vi "ziExample-ReadSingleValue.vi"(0 "Address":string="DEV", 1 "oscs/*/freq":dbl=12345.0 caption="Frequency (Hz)" format="%#_6p", 2 "demods/0/timeconstant":dbl=0.001 caption="TC (s)" format="%#_6p", 3 "phaseshift":dbl=12.0 caption="Phase (deg)" format="%#_6p", 4 "demods/0/harmonic":dbl caption="Harmonic", 5 "settingspath":string caption="Settings Path", 7 "Load":bool, 8 "Save":bool) -> (20 "Time since last boot (s)":dbl, 21 "R (Vrms)":dbl format="%#_4g", 22 "Theta (rad)":dbl, 24 "Selected Device":string)   [LabVIEW 2009]
doc: "Control a Zurich instrument device via the LabOne Labview API. \nRequirements: Zurich Instruments MFLI, HF2 or UHFLI \nExample from the Getting Started guide: A single demodulator value is read and unbundled read timestamp, X and Y.\n\n© Zurich Instruments AG, www.zhinst.com"
uses:
  <instrlib>/Zurich Instruments LabOne/Public/Data/ziTypeDemodSampleSingle.ctl
  <instrlib>/Zurich Instruments LabOne/Public/Configure/ziSetValueDoubleArray.vi
  <instrlib>/Zurich Instruments LabOne/Public/Configure/ziGetValueDouble.vi
  <instrlib>/Zurich Instruments LabOne/Public/Utility/ziTicksToS_single.vi
  <instrlib>/Zurich Instruments LabOne/Public/Configure/ziGetValueDemodSampleEx.vi
  <instrlib>/Zurich Instruments LabOne/Zurich Instruments LabOne.lvlib
panel:
  in  "stop":bool
  out "Demod Sample Out":T1={"Timestamps (ticks)"=0, "X (Vrms)"=nan, "Y (Vrms)"=nan, "Osc Phase (deg)"=nan, "Freq (Hz)"=nan, "DIO"=0, "AuxIn0 (V)"=nan, "AuxIn1 (V)"=nan, "Trigger"=0}
  out "Error Out":errorcluster
  # "This example describes how ziGetValueDemodSample.vi can be used"
  # "ziExample-ReadSingleValue.vi\nRequirements: HF2, UHFLI or MFLI\nsee block diagram for VI description"
  # "Settings"
  # "Unbundled output"
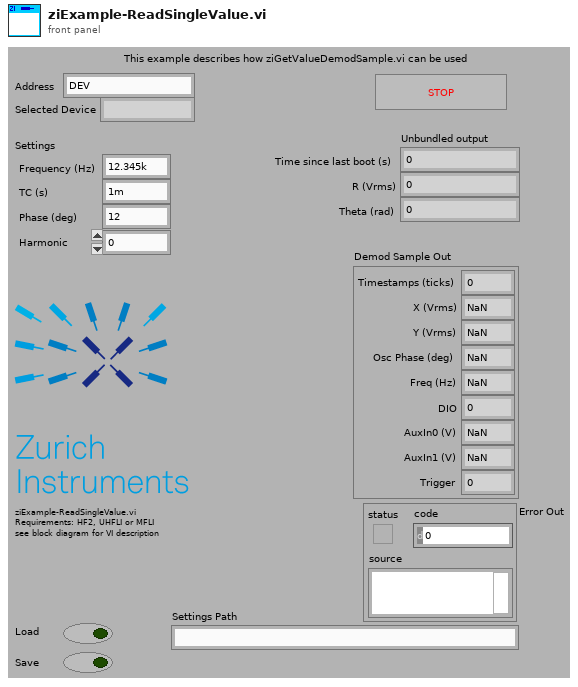
[diagram p1: front panel]
types:
  T1 = typedef "Zurich Instruments LabOne.lvlib/ziTypeDemodSampleSingle.ctl" = cluster{"Timestamps (ticks)":u64, "X (Vrms)":dbl, "Y (Vrms)":dbl, "Osc Phase (deg)":dbl, "Freq (Hz)":dbl, "DIO":u32, "AuxIn0 (V)":dbl, "AuxIn1 (V)":dbl, "Trigger":u32}
  T2 = typedef "Zurich Instruments LabOne.lvlib/ziTypeHandle.ctl" = cluster{"handleValid":bool, "Conn":u64, "Path Prefix":string, "Handle":u64, "Connected":bool, "Clockbase(s)":dbl}
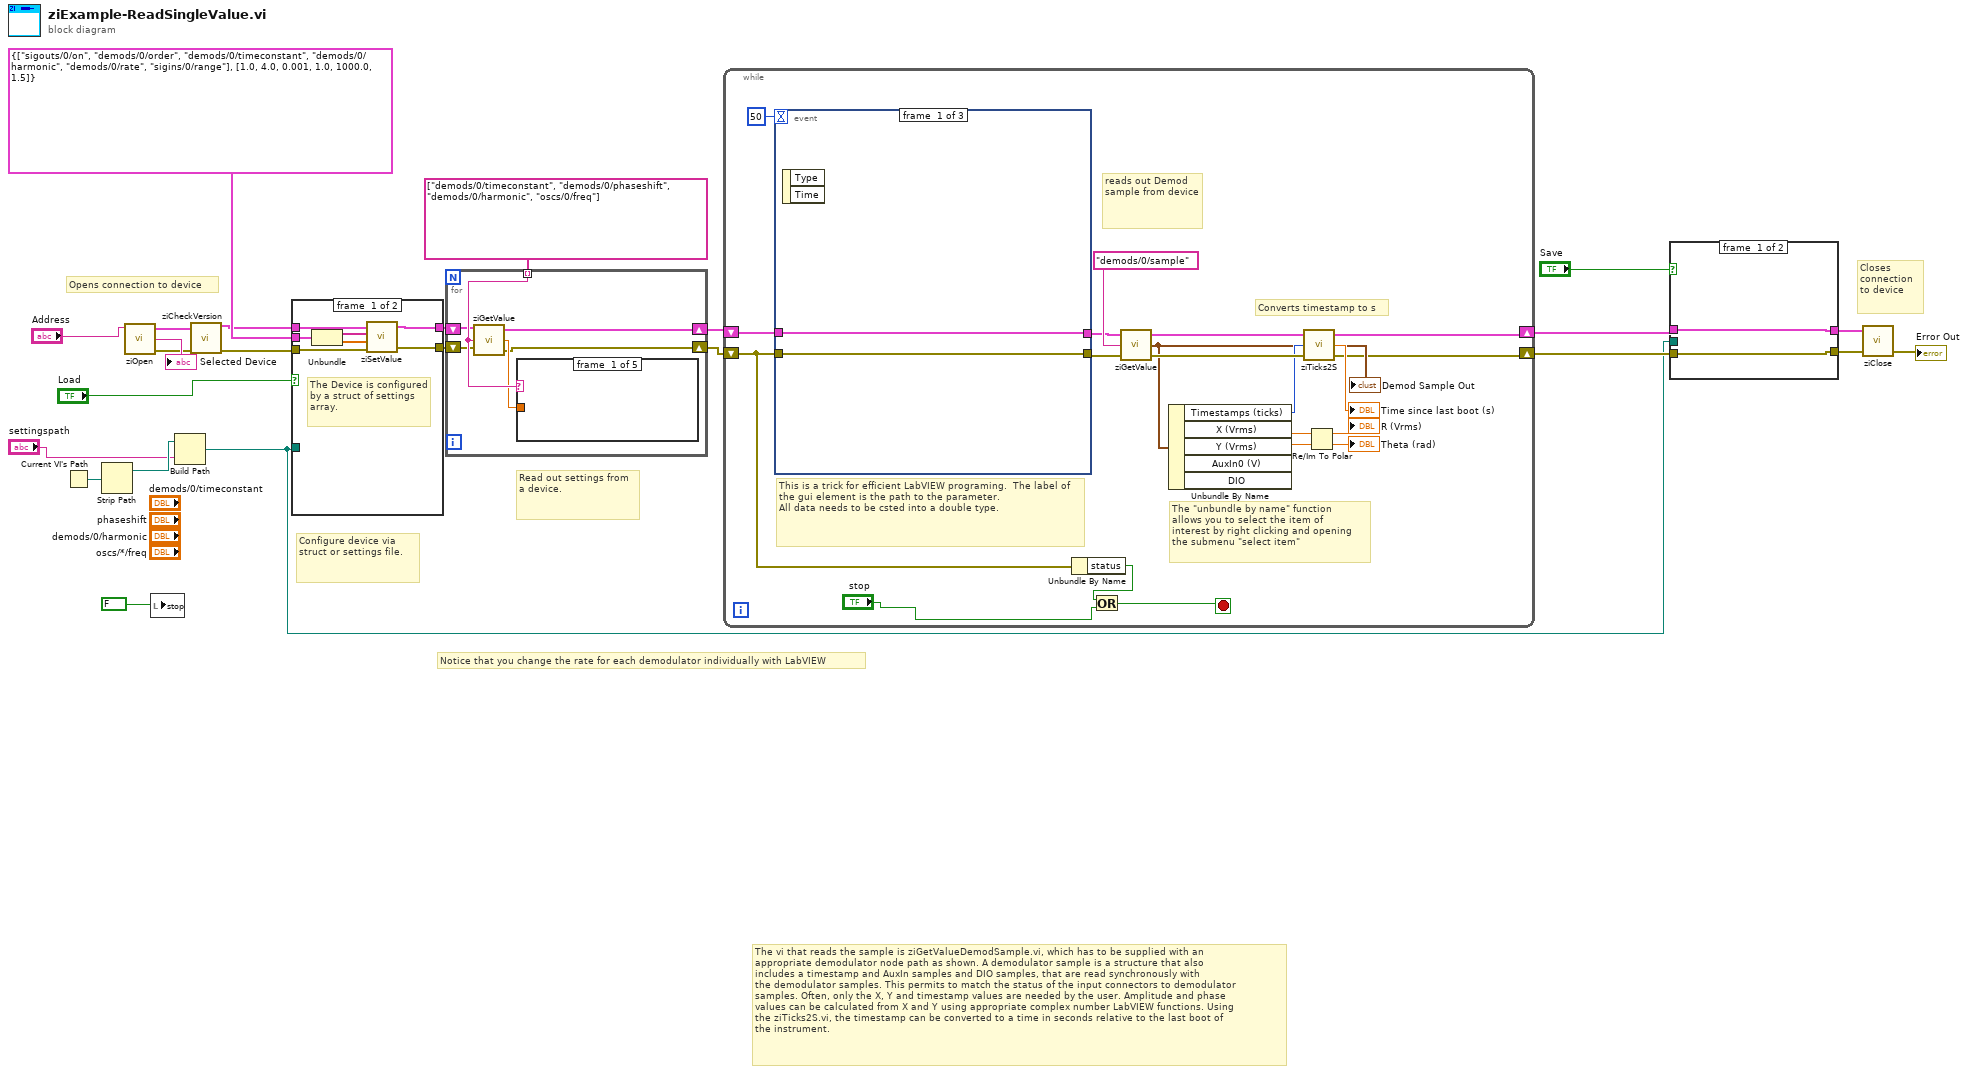
[diagram p0: block diagram]
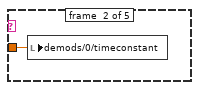
[diagram p2: hidden frame]
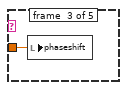
[diagram p3: hidden frame]
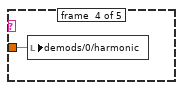
[diagram p4: hidden frame]
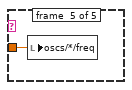
[diagram p5: hidden frame]
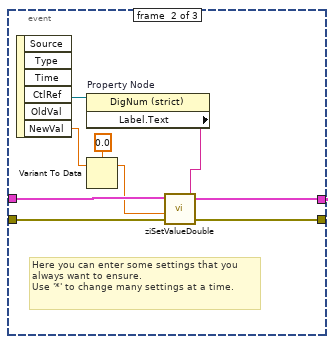
[diagram p6: hidden frame]
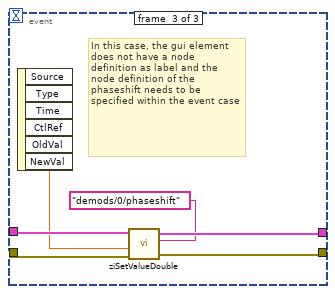
[diagram p7: hidden frame]
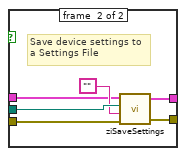
[diagram p8: hidden frame]
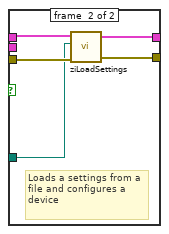
[diagram p9: hidden frame]
diagram:
  # "Closes connection to device"
  # "Opens connection to device"
  # "Read out settings from a device."
  # "Configure device via struct or settings file."
  # "Notice that you change the rate for each demodulator individually with LabVIEW"
  # "The vi that reads the sample is ziGetValueDemodSample.vi, which has to be supplied with an \nappropriate demodulator node path as shown. A demodulator sample is a structure that also \nincludes a timestamp and AuxIn samples and DIO samples, that are read synchronously with \nthe demodulator samples. This permits to match the status of the input connectors to demodulator \nsamples. Often, only the X, Y and timestamp values are needed by the user. Amplitude and phase\nvalues can be calculated from X and Y using appropriate complex number LabVIEW functions. Using \nthe ziTicks2S.vi, the timestamp can be converted to a time in seconds relative to the last boot of \nthe instrument."
  n1 = Current VI's Path() -> (path=w9:path)
  n2 = Strip Path(path=w9) -> (stripped path=w8:path)  [unwired: 1 out]
  n3 = call <instrlib>:"ziOpen.vi"("Address"="Address") -> ("Error Out"=w4:errorcluster, "Selected Device"=→"Selected Device":string, "HandleOut"=w5:T2)  [unwired: 3 in]
  n4 = local write "stop"(FALSE) -> ()
  n5 = Build Path(base path=w8, name or relative path="settingspath") -> (appended path=w6:path)
  n6 = call <instrlib>:"ziCheckVersion.vi"("Handle In"=w5, "Error In"=w4) -> ("Handle Out"=w2:T2, "Error Out"=w3:errorcluster)  [unwired: 11 in, 1 out]
  n7 = case shown="True" "Load" {
    tunnel: w3 -> [w31 w36]
    tunnel: w2 -> [w30 w33]
    tunnel: [w29 w34] -> w14
    tunnel: [w28 w35] -> w13
    tunnel: cluster{string[], dbl[]} {["sigouts/0/on", "demods/0/order", "demods/0/timeconstant", "demods/0/harmonic", "demods/0/rate", "sigins/0/range"], [1.0, 4.0, 0.001, 1.0, 1000.0, 1.5]} -> [w27 _]
    tunnel: w6 -> [_ w32]
    frame #0 {
      # "The Device is configured by a struct of settings array."
      n8 = Unbundle(w27) -> (w26:string[], w25:dbl[])
      n9 = call-poly <instrlib>:"ziSetValue.vi"("Error In"=w31, "Values"=w25, "Paths"=w26, "Handle In"=w30) -> ("Error Out"=w28:errorcluster, "Handle Out"=w29:T2)  [unwired: 1 in]
    }
    frame #1 {
      # "Loads a settings from a file and configures a device"
      n10 = call <instrlib>:"ziLoadSettings.vi"("Error in"=w36, "File path (dialog if empty)"=w32, "Handle in"=w33) -> ("Error out"=w35:errorcluster, "Handle out"=w34:T2)  [unwired: 2 in]
    }
  }
  n11 = for {
    tunnel: string[] ["demods/0/timeconstant", "demods/0/phaseshift", "demods/0/harmonic", "oscs/0/freq"] -> [w42] mode=indexing
    shift-right: [w38] -> w12
    shift-left: w14 -> [w40]
    shift-right: [w37] -> w11
    shift-left: w13 -> [w39]
    n12 = call-poly <instrlib>:"ziGetValue.vi"("error in"=w39, "Path"=w42, "Handle in"=w40) -> ("error out"=w37:errorcluster, "Value"=w41:dbl, "Handle out"=w38:T2)
    n13 = case shown="\"demods/0/timeconstant\"" w42 {
      tunnel: w41 -> [_ w43 w44 w45 w46]
      frame #0 {
      }
      frame #1 {
        n14 = local write "demods/0/timeconstant"(w43) -> ()
      }
      frame #2 {
        n15 = local write "phaseshift"(w44) -> ()
      }
      frame #3 {
        n16 = local write "demods/0/harmonic"(w45) -> ()
      }
      frame #4 {
        n17 = local write "oscs/*/freq"(w46) -> ()
      }
    }
  }
  n18 = while {
    shift-right: [w52] -> w18
    shift-left: w12 -> [w65]
    shift-right: [w51] -> w19
    shift-left: w11 -> [w49]
    stop <- w48 stop-if-true
    # "Converts timestamp to s"
    # "reads out Demod sample from device"
    # "This is a trick for efficient LabVIEW programing.  The label of the gui element is the path to the parameter.\nAll data needs to be csted into a double type."
    # "The \"unbundle by name\" function\nallows you to select the item of \ninterest by right clicking and opening\nthe submenu \"select item\""
    n19 = event shown="[1] \"oscs/*/freq\", \"demods/0/harmonic\", \"demods/0/timeconstant\": Value Change" {
      selector: _ -> [_ _ _]
      dyn-events: _ -> [_ _ _]
      timeout: 50 -> [_ _ _]
      tunnel: w65 -> [w68 w75 w82]
      tunnel: w49 -> [w67 w72 w81]
      tunnel: [w68 w74 w83] -> w53
      tunnel: [w67 w73 w80] -> w54
      event #0 {
        n20 = event-data() -> ()  [unwired: 3 out]
      }
      event #1 {
        # "Here you can enter some settings that you always want to ensure.\nUse '*' to change many settings at a time."
        n21 = event-data() -> ("CtlRef"=w77:refnum<vi>, "NewVal"=w76:dbl)  [unwired: 5 out]
        n22 = property on="Property Node" class="DigNum (strict)"(reference=w77) -> ("Label.Text"=w69:string)  [unwired: 1 in, 2 out]
        n23 = Variant To Data(Variant=w76, type=0.0 ("demods/")) -> (data=w71:dbl)  [unwired: 1 in, 1 out]
        n24 = call <instrlib>:"ziSetValueDouble.vi"("Error In"=w72, "Value"=w71, "Path"=w69, "Handle In"=w75) -> ("Error Out"=w73:errorcluster, "Handle Out"=w74:T2)  [unwired: 1 out]
      }
      event #2 {
        # "In this case, the gui element does not have a node definition as label and the node definition of the phaseshift needs to be\nspecified within the event case"
        n25 = event-data() -> ("NewVal"=w78:dbl)  [unwired: 6 out]
        n26 = call <instrlib>:"ziSetValueDouble.vi"("Error In"=w81, "Value"=w78, "Path"="demods/0/phaseshift", "Handle In"=w82) -> ("Error Out"=w80:errorcluster, "Handle Out"=w83:T2)  [unwired: 1 out]
      }
    }
    n27 = Unbundle By Name(w49) -> ("status"=w50:bool)
    n28 = Or(x=w50, y="stop") -> (x .or. y?=w48:bool)
    n29 = call-poly <instrlib>:"ziGetValue.vi"("error in"=w54, "Path"="demods/0/sample", "Handle In"=w53) -> ("error out"=w64:errorcluster, "Demod Sample Out"=w59:T1, "Handle Out"=w63:T2)
    "Demod Sample Out" <- w59
    n30 = Unbundle By Name(w59) -> ("Timestamps (ticks)"=w61:u64, "X (Vrms)"=w55:dbl, "Y (Vrms)"=w56:dbl)  [unwired: 2 out]
    n31 = call-poly <instrlib>:"ziTicks2S.vi"("Error In"=w64, "Timestamp(ticks)"=w61, "Handle In"=w63) -> ("Error Out"=w51:errorcluster, "Timestamp(s)"=→"Time since last boot (s)":dbl, "Handle Out"=w52:T2)
    n32 = Re/Im To Polar(2:w56, 3:w55) -> (0:→"Theta (rad)":dbl, 1:→"R (Vrms)":dbl)
  }
  n33 = case shown="True" "Save" {
    tunnel: [w84 w90] -> w22
    tunnel: [w85 w89] -> w21
    tunnel: w6 -> [_ w91]
    tunnel: w19 -> [w85 w87]
    tunnel: w18 -> [w84 w86]
    frame #0 {
    }
    frame #1 {
      # "Save device settings to\na Settings File"
      n34 = call <instrlib>:"ziSaveSettings.vi"("Error In"=w87, "Path (\"\")"="", "file path (dialog if empty)"=w91, "Handle In"=w86) -> ("Error Out"=w89:errorcluster, "Handle Out"=w90:T2)  [unwired: 1 out]
    }
  }
  n35 = call <instrlib>:"ziClose.vi"("Error In"=w21, "Handle In"=w22) -> ("Error Out"=→"Error Out":errorcluster)  [unwired: 2 in, 1 out]
